vi "P3_1_Graficas.vi"() -> ()   [LabVIEW 2020]
panel:
  out "Grafico temperatura y filtro EMA":dynamicdata(graph)
  in  "stop":bool
  out "appended array":dbl[][](array[numeric])
  out "min value":dbl
  out "max value":dbl
  out "Waveform Graph 2":dbl[](graph)
  out "Waveform Graph":dbl[](graph)
  out "EMA":dbl[](array[numeric])
  out "fahrenheit":dbl[](array[numeric])
  out "celcius":dbl[](array[numeric])
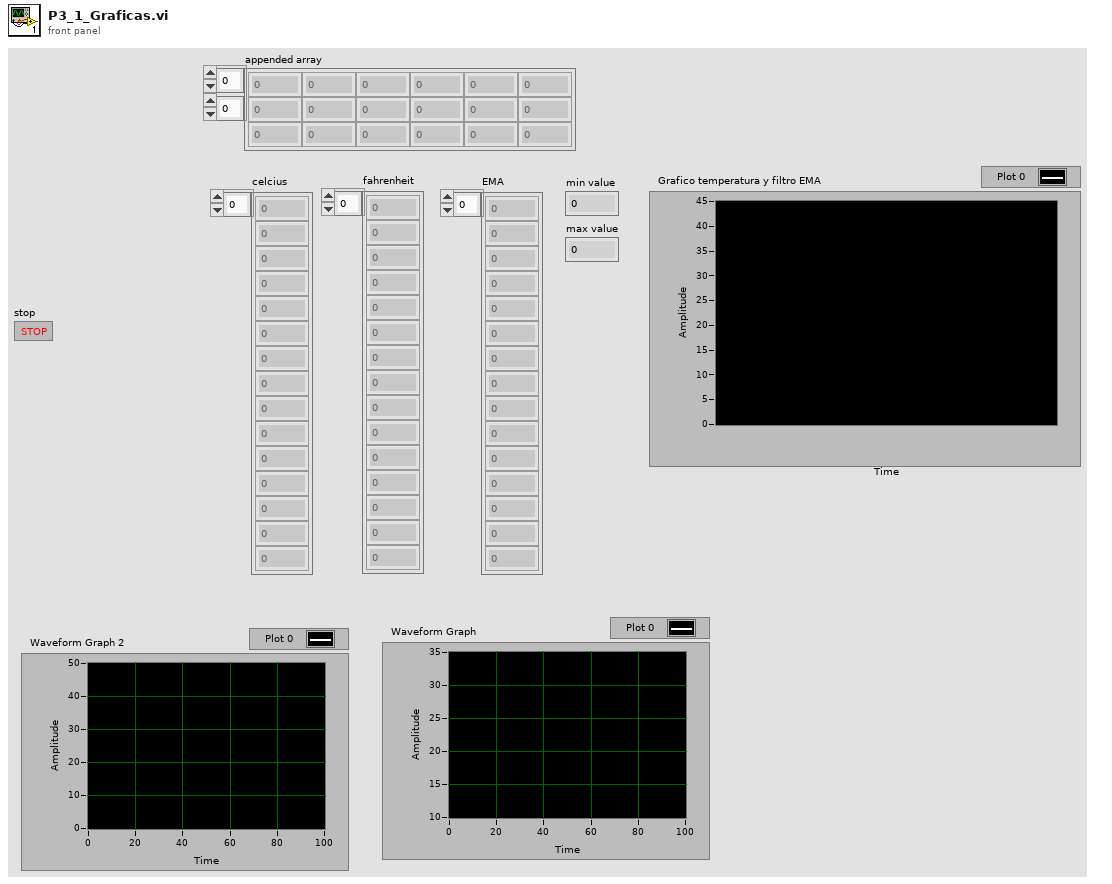
[diagram p1: front panel]
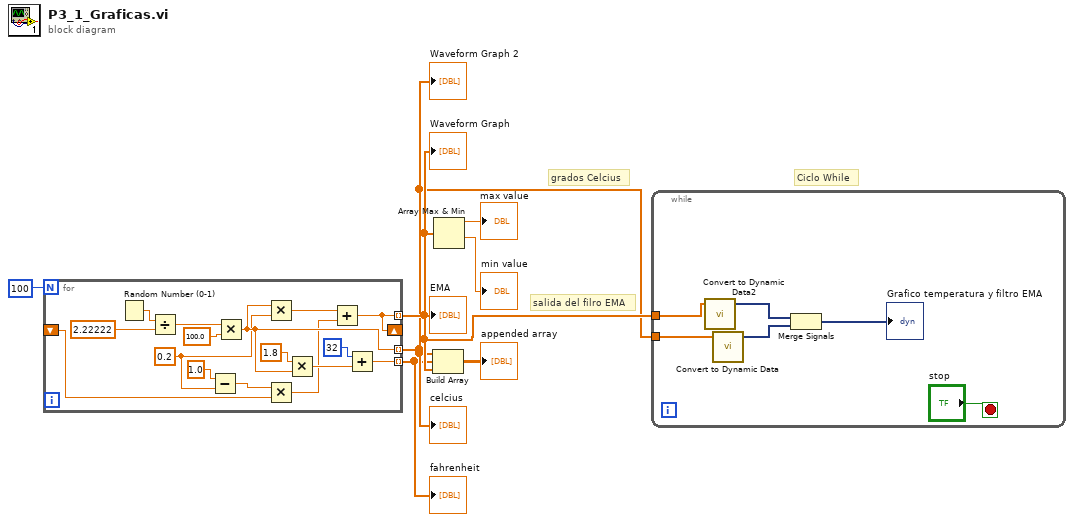
[diagram p0: block diagram]
diagram:
  # "Ciclo While"
  # "grados Celcius"
  # "salida del filro EMA"
  n1 = for {
    N: 100 -> [_]
    tunnel: [w15] -> w2 mode=indexing
    tunnel: [w16] -> w1 mode=indexing
    shift-right: [w9] -> _
    shift-left: _ -> [w8]
    tunnel: [w9] -> w3 mode=indexing
    w13 = 0.2
    n2 = Random Number (0-1)() -> (number: 0 to 1=w23:dbl)
    n3 = Divide(x=w23, y=2.22222) -> (x/y=w20:dbl)
    n4 = Subtract(x=1.0, y=w13) -> (x-y=w11:dbl)
    n5 = Multiply(x=w20, y=100.0 ("x*y")) -> (x*y=w15:dbl)
    n6 = Multiply(x=w15, y=w13) -> (x*y=w10:dbl)
    n7 = Multiply(x=w11, y=w8) -> (x*y=w12:dbl)
    n8 = Multiply(x=1.8, y=w15) -> (x*y=w18:dbl)
    n9 = Add(x=w10, y=w12) -> (x+y=w9:dbl)
    n10 = Add(x=32, y=w18) -> (x+y=w16:dbl)
  }
  "celcius" <- w2
  "fahrenheit" <- w1
  "EMA" <- w3
  "Waveform Graph" <- w3
  "Waveform Graph 2" <- w2
  n11 = Build Array(w2, w1, w3) -> (→"appended array":dbl[][])
  n12 = Array Max & Min(array=w3) -> (max value=→"max value":dbl, min value=→"min value":dbl)  [unwired: 2 out]
  n13 = while {
    tunnel: w2 -> [w25]
    tunnel: w3 -> [w24]
    stop <- "stop" stop-if-true
    n14 = call "Convert to Dynamic Data2"("Array"=w24) -> ("Dynamic Data Type"=w27:dynamicdata)  [unwired: 3 in]
    n15 = call "Convert to Dynamic Data"("Array"=w25) -> ("Dynamic Data Type"=w26:dynamicdata)  [unwired: 3 in]
    n16 = Merge Signals "Merge Signals"(w27, w26) -> (→"Grafico temperatura y filtro EMA":dynamicdata)
  }
